vi "Save FITS coop.vi"(6 "Save to FITS?":bool, 8 "error in (no error)":errorcluster, 9 "FITS /UI in":T1={"Wavelength (nm)"=530.15, "Exposure (s)"=0.05, "Tuning Delay (ms)"=200.0, "Beam Type (-1/1)"=1.0, "Tuning Voltages"=[1.111, 2.222, 3.333, 4.444], "Observer"="observer", "Light Shapping Diffuser"=enum."In Beam", "Comment"="", "Data Type"=enum."LIVE", "Mod Cycles"=1, "SCD Calibration Optics"=enum."1 - Polarizer @0, I+Q", "SCD Emission Line Filter"=enum."1-557.6nm", "Cookbook"="", "COMP-S Calibration Wheel"=enum."Dark", "COMP-S Andover Filter Wheel"=enum."530.3nm/HWB 0.34nm (Fe XIV)", "FOV Rotation (deg)"=66.0, "Objective Lens Position (mm)"=0.0, "Occulter size"=0.0, "Time End"=timestamp(3382374145.421875 s since 1904-01-01), "Acc Exposure (s)"=0.0, "Time Stamp Array"=[], "Camera Serial Number"=[], "Camera Temp"=[], "Camera PI (mm)"=[0.0, 0.0, 0.0], "Time Start"=timestamp(3382374145.421875 s since 1904-01-01), "Peripherals"={"ILX controler"=FALSE, "Zone temperatures"=FALSE, "Andor"=FALSE, "Andor 2"=FALSE, "PI Stages"=FALSE, "AISAS mechanisms"=FALSE, "AISAS Mech.lvclass"=refnum, "Zone temp ref"=variant, "FWs"=FALSE}, "FITS paths"=[], "Cameras"=enum."Andor", "load preset cbk"=FALSE, "periodic check count"=0, "COMP-S Calibration Wheel 2"=enum."Dark", "Calib"=enum."Dark", "Abso Aperture"=66.0, "Nominal Aperture"=66.0} {"Nominal Aperture" format="%.1f"; "Abso Aperture" format="%.1f"; "Camera PI (mm)" format="%_3g"; "Acc Exposure (s)" format="%^.3g"; "Occulter size" format="%.2f"; "Objective Lens Position (mm)" min=70.0 max=152.0 format="%.2f"; "FOV Rotation (deg)" format="%.1f"; "Exposure (s)" format="%^.3g"; "Wavelength (nm)" format="%_6g"}, 10 "Image Data":u16[][](array[numeric]), 11 "Camera in":refnum<class "Camera.lvclass">) -> (0 "error out":errorcluster, 1 "FITS /UI out":T1={"Wavelength (nm)"=530.15, "Exposure (s)"=0.05, "Tuning Delay (ms)"=200.0, "Beam Type (-1/1)"=1.0, "Tuning Voltages"=[1.111, 2.222, 3.333, 4.444], "Observer"="observer", "Light Shapping Diffuser"=enum."In Beam", "Comment"="", "Data Type"=enum."LIVE", "Mod Cycles"=1, "SCD Calibration Optics"=enum."1 - Polarizer @0, I+Q", "SCD Emission Line Filter"=enum."1-557.6nm", "Cookbook"="", "COMP-S Calibration Wheel"=enum."Dark", "COMP-S Andover Filter Wheel"=enum."530.3nm/HWB 0.34nm (Fe XIV)", "FOV Rotation (deg)"=66.0, "Objective Lens Position (mm)"=0.0, "Occulter size"=0.0, "Time End"=timestamp(3382374145.421875 s since 1904-01-01), "Acc Exposure (s)"=0.0, "Time Stamp Array"=[], "Camera Serial Number"=[], "Camera Temp"=[], "Camera PI (mm)"=[0.0, 0.0, 0.0], "Time Start"=timestamp(3382374145.421875 s since 1904-01-01), "Peripherals"={"ILX controler"=FALSE, "Zone temperatures"=FALSE, "Andor"=FALSE, "Andor 2"=FALSE, "PI Stages"=FALSE, "AISAS mechanisms"=FALSE, "AISAS Mech.lvclass"=refnum, "Zone temp ref"=variant, "FWs"=FALSE}, "FITS paths"=[], "Cameras"=enum."Andor", "load preset cbk"=FALSE, "periodic check count"=0, "COMP-S Calibration Wheel 2"=enum."Dark", "Calib"=enum."Dark", "Abso Aperture"=66.0, "Nominal Aperture"=66.0} {"Nominal Aperture" format="%.1f"; "Abso Aperture" format="%.1f"; "Camera PI (mm)" format="%_3g"; "Acc Exposure (s)" format="%^.3g"; "Occulter size" format="%.2f"; "Objective Lens Position (mm)" min=70.0 max=152.0 format="%.2f"; "FOV Rotation (deg)" format="%.1f"; "Exposure (s)" format="%^.3g"; "Wavelength (nm)" format="%_6g"}, 2 "Image Data out":u16[][](array[numeric]), 3 "Camera out":refnum<class "Camera.lvclass">)   [LabVIEW 2014]
uses:
  Camera/Camera/Camera.lvclass
  Controls/SCD - FITS Cluster.ctl
  AISAS/Mech/AISAS Mech.lvclass
  AISAS/Controls/Diffuser.ctl
  Controls/FITS Data type.ctl
  Controls/SCD - Calibration Optics Filter Wheel.ctl
  Controls/SCD - EDT - Emission Line Filter Wheel.ctl
  Controls/CoMP-S Controls/Polarization Optics Filter Wheel.ctl
  Controls/CoMP-S Controls/Emission Line Filter Wheel.ctl
  AISAS/Controls/focus.ctl
  Controls/peripherals.ctl
  Controls/Cameras select.ctl
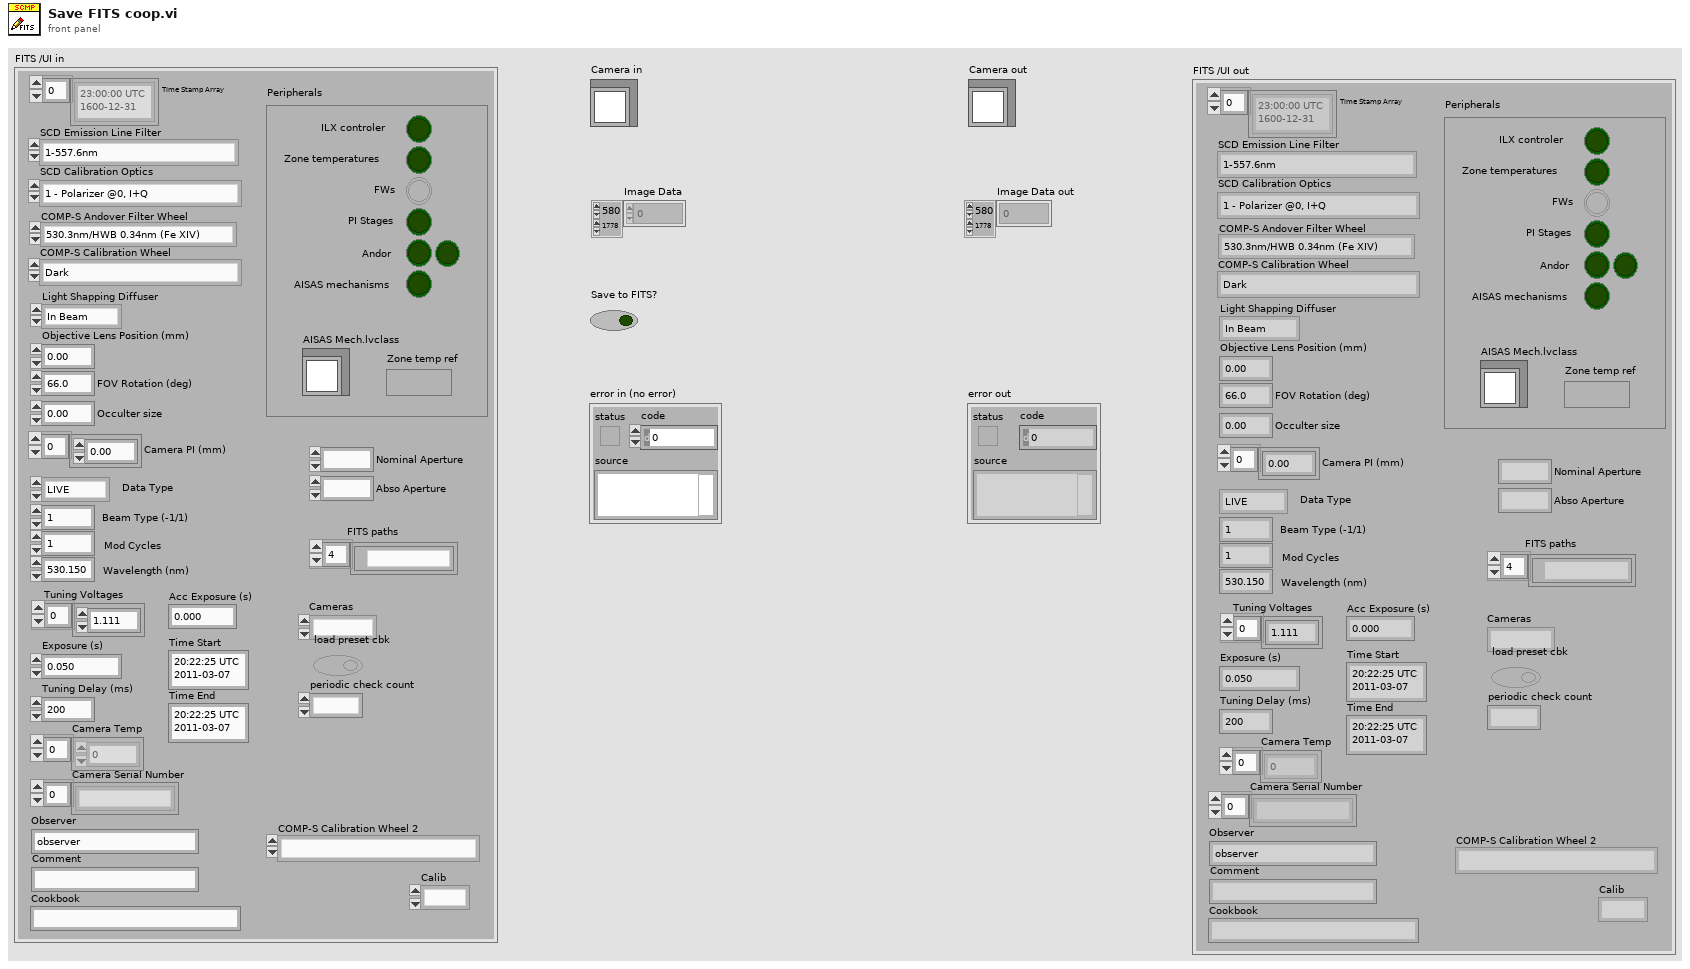
[diagram p1: front panel]
types:
  T1 = typedef "SCD - FITS Cluster.ctl" = cluster{"Wavelength (nm)":dbl, "Exposure (s)":dbl, "Tuning Delay (ms)":dbl, "Beam Type (-1/1)":dbl, "Tuning Voltages":dbl[], "Observer":string, "Light Shapping Diffuser":T2, "Comment":string, "Data Type":T3, "Mod Cycles":u16, "SCD Calibration Optics":T4, "SCD Emission Line Filter":T5, "Cookbook":string, "COMP-S Calibration Wheel":T6, "COMP-S Andover Filter Wheel":T7, "FOV Rotation (deg)":dbl, "Objective Lens Position (mm)":T8, "Occulter size":dbl, "Time End":timestamp, "Acc Exposure (s)":dbl, "Time Stamp Array":timestamp[], "Camera Serial Number":string[], "Camera Temp":dbl[], "Camera PI (mm)":dbl[], "Time Start":timestamp, "Peripherals":T9, "FITS paths":path[], "Cameras":T10, "load preset cbk":bool, "periodic check count":i32, "COMP-S Calibration Wheel 2":T6, "Calib":enum16{"Dark", "Flat"}, "Abso Aperture":dbl, "Nominal Aperture":dbl}
  T2 = typedef "Diffuser.ctl" = enum16{"Out of Beam", "In Beam"}
  T3 = typedef "FITS Data type.ctl" = enum16{"LIVE", "DARK", "FLAT", "CALI", "OBSE", "ABSO", "AURE", "TARG", "OBJE", "HOLE", "OREX", "THRO", "CHIP"}
  T4 = typedef "SCD - Calibration Optics Filter Wheel.ctl" = enum16{"1 - Polarizer @0, I+Q", "2 - Polarizer @90, I-Q", "3 - Polarizer @45, I+U", "4 - Polarizer @135, I-U", "5 - Polarizer @0, Retarder @45, I+V", "6 - Polarizer @0, Retarder @135, I-V", "7 - Dark", "8 - Clear", "9 - N/A"}
  T5 = typedef "SCD - EDT - Emission Line Filter Wheel.ctl" = enum16{"1-557.6nm", "2-587.6nm", "3-589.6nm", "4-630.2nm", "5-656.4nm", "6-849.8nm", "7-854.2nm", "8-866.2nm", "9-1083.0nm"}
  T6 = typedef "Polarization Optics Filter Wheel.ctl" = enum16{"Dark", "Clear", "Exchange Lens", "Polarizer @0, I+Q", "Polarizer @90, I-Q", "Polarizer @45, I+U", "Polarizer @135, I-U", "Polarizer @0, Retarder @45, I+V", "Polarizer @0, Retarder @135, I-V"}
  T7 = typedef "Emission Line Filter Wheel.ctl" = enum16{"530.3nm/HWB 0.34nm (Fe XIV)", "587.6nm/HBW 0.44nm (He I D3)", "637.5nm/HBW 0.53nm (Fe X)", "656.3nm/HBW 0.57nm (H-Alpha)", "789.2nm/HBW 0.85nm (Fe XI)", "854.2nm/HBW 1.01nm (Ca I)", "1074.7nm/HBW 2.34nm (Fe XIII)", "1079.8nm/HBW 1.64nm (Fe XIII)", "1083.0nm/HBW 1.66nm (He I)"}
  T8 = typedef "focus.ctl" = dbl
  T9 = typedef "peripherals.ctl" = cluster{"ILX controler":bool, "Zone temperatures":bool, "Andor":bool, "Andor 2":bool, "PI Stages":bool, "AISAS mechanisms":bool, "AISAS Mech.lvclass":refnum<class "AISAS Mech.lvclass">, "Zone temp ref":variant, "FWs":bool}
  T10 = typedef "Cameras select.ctl" = enum16{"Andor", "GDR"}
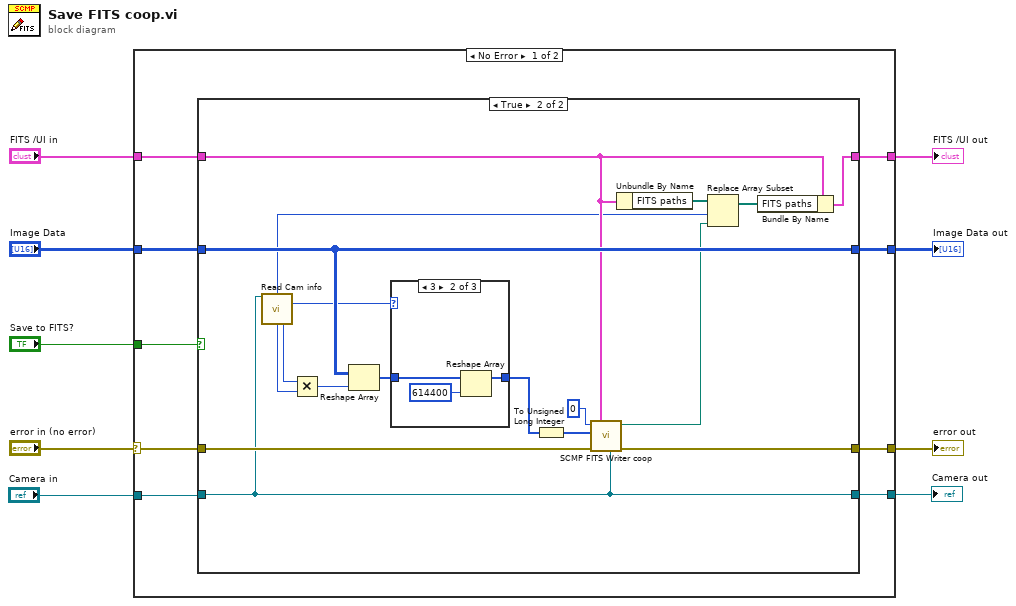
[diagram p0: block diagram]
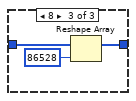
[diagram p4: hidden frame]
diagram:
  n1 = case shown="No Error" "error in (no error)" {
    selector: "error in (no error)" -> [w16 w51]
    tunnel: [w15 w51] -> w8
    tunnel: [w10 w50] -> w6
    tunnel: "Camera in" -> [w11 w50]
    tunnel: [w18 w49] -> w5
    tunnel: "FITS /UI in" -> [w17 w49]
    tunnel: "Save to FITS?" -> [w14 _]
    tunnel: "Image Data" -> [w13 w48]
    tunnel: [w12 w48] -> w1
    frame No Error {
      n2 = case shown="True" w14 {
        tunnel: w13 -> [w20 w35]
        tunnel: w16 -> [w22 w40]
        tunnel: [w22 w39] -> w15
        tunnel: [w21 w30] -> w18
        tunnel: w17 -> [w21 w32]
        tunnel: [w20 w35] -> w12
        tunnel: w11 -> [w19 w25]
        tunnel: [w19 w25] -> w10
        frame False {
        }
        frame True {
          n3 = call-dynamic "Read Cam info.vi"("Camera in"=w25) -> ("Idx"=w24:i32, "BDiv"=w26:u8, "AOI Width"=w29:i32, "AOI Height"=w28:i32)  [unwired: 5 in, 6 out]
          n4 = Multiply(x=w28, y=w29) -> (x*y=w27:i32)
          n5 = Reshape Array(w35, w27) -> (w37:u16[])
          n6 = case shown="3" w26 {
            tunnel: w37 -> [w41 w44 w46]
            tunnel: [w41 w43 w45] -> w36
            frame 1, Default {
            }
            frame 3 {
              n7 = Reshape Array(w44, 614400 ("dimension size")) -> (w43:u16[])
            }
            frame 8 {
              n8 = Reshape Array(w46, 86528 ("dimension size")) -> (w45:u16[])
            }
          }
          n9 = To Unsigned Long Integer(number=w36) -> (unsigned 32bit integer=w23:u32[])
          n10 = call "SCMP FITS Writer coop.vi"("Camera.lvclass"=w25, "FITS Cluster"=w32, "error in"=w40, "Image Vector"=w23, "Wavelength (0..n)"=0) -> ("error out"=w39:errorcluster, "Current FITS Path"=w33:path)  [unwired: 5 in]
          n11 = Unbundle By Name(w32) -> ("FITS paths"=w34:path[])
          n12 = Replace Array Subset(array=w34, new element=w33, index=w24) -> (w31:path[])
          n13 = Bundle By Name(cluster=w32, "FITS paths"=w31) -> (w30:T1)
        }
      }
    }
    frame Error {
    }
  }
  "error out" <- w8
  "Camera out" <- w6
  "FITS /UI out" <- w5
  "Image Data out" <- w1
